vi "Standard Event Status Enable.vi"(0 "VISA resource name":refnum<visa-resource-name>, 5 "Standard Event Status Enable":T1, 11 "error in (no error)":errorcluster) -> (4 "VISA resource name out":refnum<visa-resource-name>, 15 "error out":errorcluster)   [LabVIEW 2018, in "XP Power PLS600.lvlib"]
doc: "Enables the events for which the status is to be monitored in the instrument.\n\nThe Standard Event Register consists of the following 8 bits.\n\nBIT 0: Operation Complete\nBIT 1: Request Control\nBIT 2: Query Error\nBIT 3: Device Dependant Error\nBIT 4: Execution Error\nBIT 5: Command Error\nBIT 6: User Request\nBIT 7: Power On"
uses:
  XP Power PLS600.lvlib
panel:
  # "BIT 0: Operation Complete\nBIT 1: Request Control\nBIT 2: Query Error\nBIT 3: Device Dependant Error\nBIT 4: Execution Error\nBIT 5: Command Error\nBIT 6: User Request\nBIT 7: Power On"
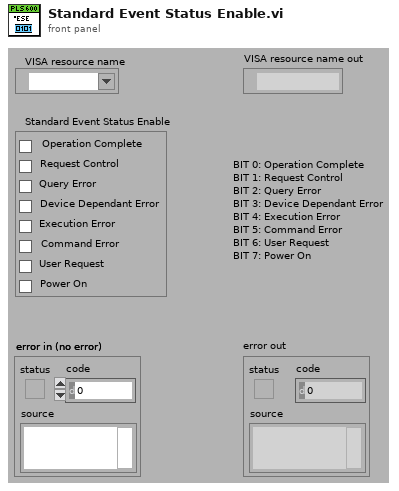
[diagram p1: front panel]
types:
  T1 = cluster{"Operation Complete":bool, "Request Control":bool, "Query Error":bool, "Device Dependant Error":bool, "Execution Error":bool, "Command Error":bool, "User Request":bool, "Power On":bool}
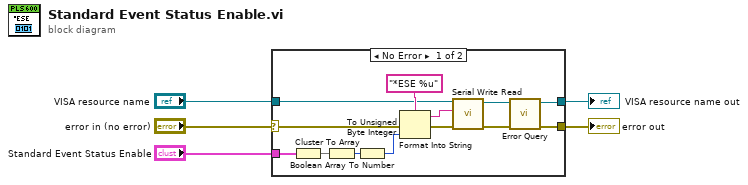
[diagram p0: block diagram]
diagram:
  n1 = case shown="No Error" "error in (no error)" {
    selector: "error in (no error)" -> [w18 w20]
    tunnel: "VISA resource name" -> [w8 w19]
    tunnel: [w6 w19] -> w5
    tunnel: [w9 w20] -> w4
    tunnel: "Standard Event Status Enable" -> [w15 _]
    frame No Error {
      n2 = Cluster To Array(cluster=w15) -> (array=w16:bool[])
      n3 = Boolean Array To Number(Boolean array=w16) -> (number=w14:u32)
      n4 = To Unsigned Byte Integer(number=w14) -> (unsigned 8bit integer=w13:u8)
      n5 = Format Into String(format string="*ESE %u" ("Command to Send"), error in=w18, w13) -> (resulting string=w7:string, error out=w10:errorcluster)  [unwired: 1 in]
      n6 = call "Serial Write Read.vi"("error in (no error)"=w10, "Write Buffer"=w7, "VISA resource name"=w8) -> ("error out"=w12:errorcluster, "VISA resource name out"=w11:refnum<visa-resource-name>)  [unwired: 6 in, 1 out]
      n7 = call "Error Query.vi"("error in (no error)"=w12, "VISA resource name"=w11) -> ("error out"=w9:errorcluster, "VISA resource name out"=w6:refnum<visa-resource-name>)  [unwired: 6 in, 2 out]
    }
    frame Error {
    }
  }
  "error out" <- w4
  "VISA resource name out" <- w5
